vi "SIM Integrator init (for core) (vector).vi"(6 "Block Tag":string, 9 "IC":dbl[](array[numeric]), 10 "Width":i32, 11 "Registry In":T1) -> (0 "error out":i32, 3 "Registry Out":T1)   [LabVIEW 2020]
uses:
  SIM Simulation Registry.ctl
  SIM Registry Node Header.ctl
  SIM Registry Node Record.ctl
  SIM trigger type.ctl
  SIM solver state data.ctl
  SIM limit type.ctl
  SIM discrete data.ctl
  SIM Discrete state data.ctl
  SIM Simulation Registry Error.ctl
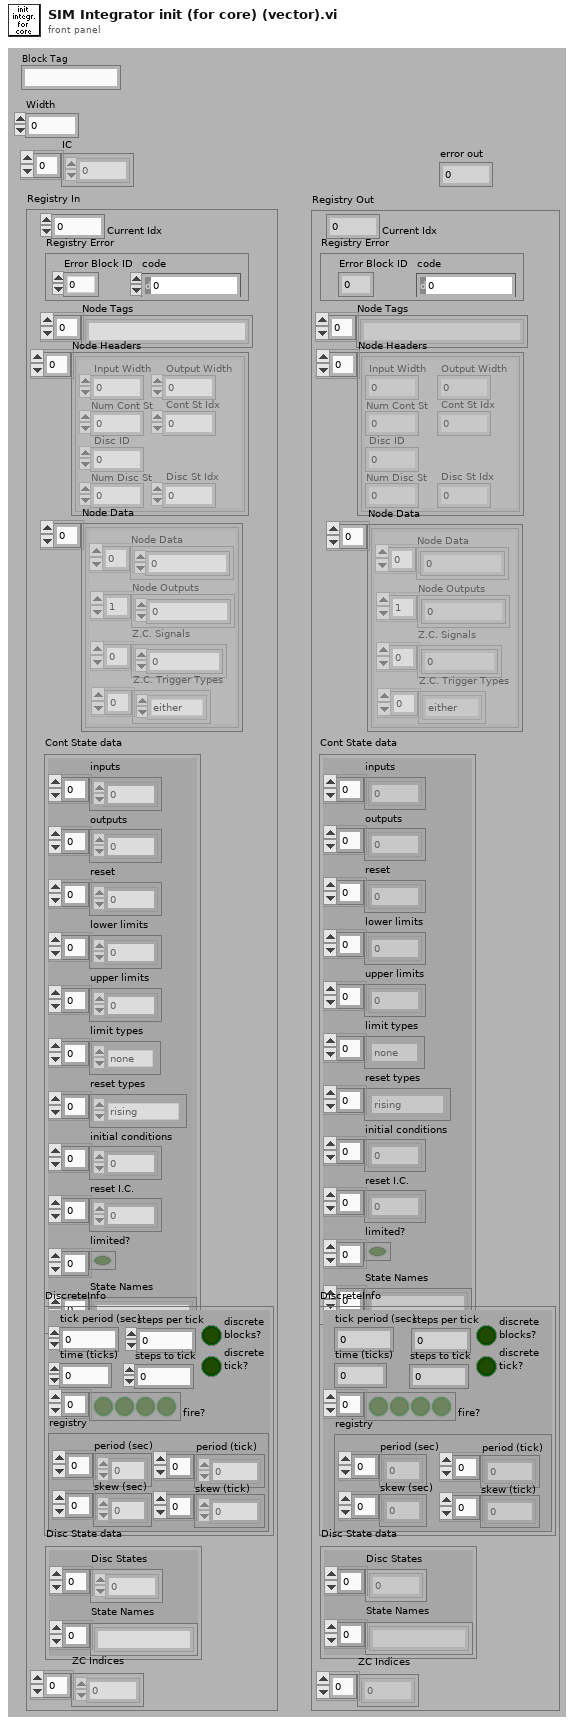
[diagram p1: front panel]
types:
  T1 = typedef "SIM Simulation Registry.ctl" = cluster{"Current Idx":i32, "Node Tags":string[], "Node Headers":T2[], "Node Data":T3[], "Cont State data":T5, "DiscreteInfo":T7, "Disc State data":T8, "Registry Error":T9, "ZC Indices":i32[]}
  T2 = typedef "SIM Registry Node Header.ctl" = cluster{"Input Width":i32, "Disc ID":i32, "Num Cont St":i32, "Cont St Idx":i32, "Num Disc St":i32, "Disc St Idx":i32, "Output Width":i32}
  T3 = typedef "SIM Registry Node Record.ctl" = cluster{"Node Data":dbl[], "Node Outputs":dbl[], "Z.C. Signals":dbl[], "Z.C. Trigger Types":T4[]}
  T4 = typedef "SIM trigger type.ctl" = enum16{"rising", "falling", "either", "none"}
  T5 = typedef "SIM solver state data.ctl" = cluster{"inputs":dbl[], "outputs":dbl[], "reset":dbl[], "lower limits":dbl[], "upper limits":dbl[], "limit types":T6[], "reset types":T4[], "initial conditions":dbl[], "reset I.C.":dbl[], "limited?":bool[], "State Names":string[]}
  T6 = typedef "SIM limit type.ctl" = enum16{"upper", "lower", "both", "none"}
  T7 = typedef "SIM discrete data.ctl" = cluster{"tick period (sec)":dbl, "time (ticks)":i32, "fire?":bool[], "registry":cluster{"period (sec)":dbl[], "skew (sec)":dbl[], "period (tick)":i32[], "skew (tick)":i32[]}, "discrete \nblocks?":bool, "steps per tick":dbl, "steps to tick":dbl, "discrete \ntick?":bool}
  T8 = typedef "SIM Discrete state data.ctl" = cluster{"Disc States":dbl[], "State Names":string[]}
  T9 = typedef "SIM Simulation Registry Error.ctl" = cluster{"Error Block ID":i32, "code":i32}
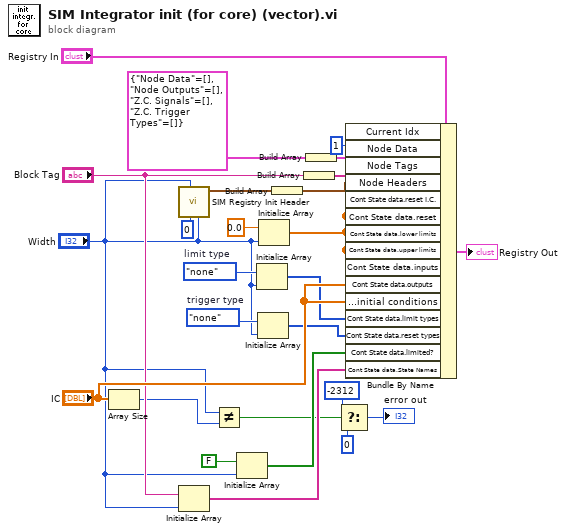
[diagram p0: block diagram]
diagram:
  w26 = SIM_trigger_type."none"  # trigger type
  w25 = SIM_limit_type."none"  # limit type
  n1 = Array Size(array="IC") -> (size(s)=w1:i32)
  n2 = call "SIM Registry Init Header.vi"("Num Cont States"="Width", "State Idx"=0, "Input Width"="Width") -> ("Node Header"=w9:T2)  [unwired: 5 in, 3 out]
  n3 = Initialize Array("Block Tag", "Width") -> (w14:string[])
  n4 = Not Equal?(x="Width", y=w1) -> (x != y?=w12:bool)
  n5 = Initialize Array(FALSE, "Width") -> (w15:bool[])
  n6 = Initialize Array(w25, "Width") -> (w18:T6[])
  n7 = Initialize Array(w26, "Width") -> (w17:T4[])
  n8 = Initialize Array(0.0 ("limited signal"), "Width") -> (w20:dbl[])
  n9 = Build Array(w9) -> (w8:T2[])
  n10 = Build Array("Block Tag") -> (w5:string[])
  n11 = Build Array(T3 {"Node Data"=[], "Node Outputs"=[], "Z.C. Signals"=[], "Z.C. Trigger Types"=[]} ("Node Record")) -> (w7:T3[])
  n12 = Select(t=-2312 ("error.code"), s=w12, f=0) -> (s? t:f=→"error out":i32)
  n13 = Bundle By Name(cluster="Registry In", "Current Idx"=1, "Node Data"=w7, "Node Tags"=w5, "Node Headers"=w8, "Cont State data.reset I.C."=w20, "Cont State data.reset"=w20, "Cont State data.lower limits"=w20, "Cont State data.upper limits"=w20, "Cont State data.inputs"=w20, "Cont State data.outputs"="IC", "Cont State data.initial conditions"="IC", "Cont State data.limit types"=w18, "Cont State data.reset types"=w17, "Cont State data.limited?"=w15, "Cont State data.State Names"=w14) -> (→"Registry Out":T1)
